vi "Main VI open close.vi"() -> ()   [LabVIEW 2022 SP3]
panel:
  in  "stop":bool
  in  "GO Button":bool
  in  "Enum":enum16{"SUBVI1", "SUBVI2", "SUBVI3"}(ring)
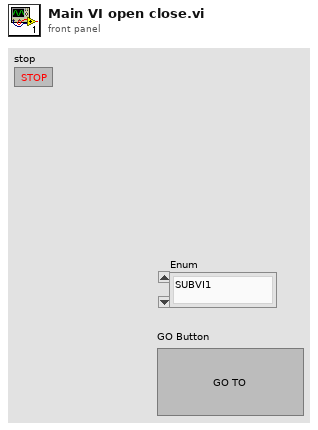
[diagram p1: front panel]
types:
  T1 = enum32{"Invalid", "Standard", "Closed", "Hidden", "Minimized", "Maximized"}
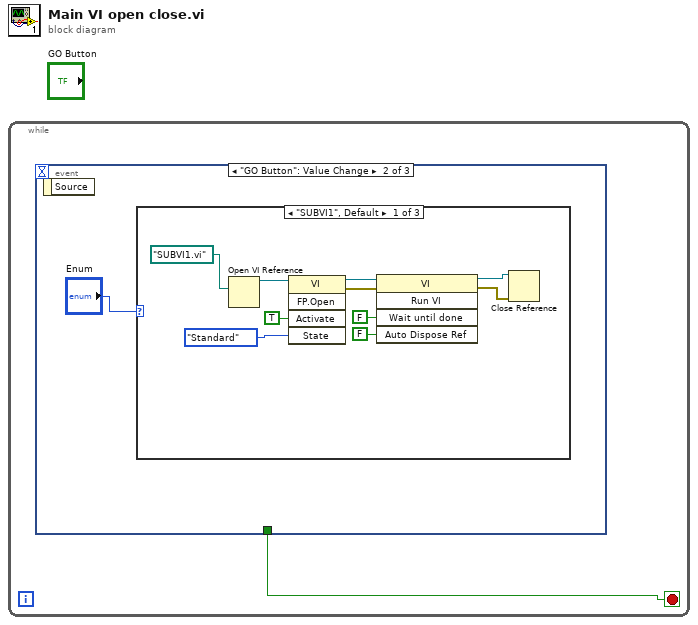
[diagram p0: block diagram]
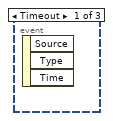
[diagram p2: hidden frame]
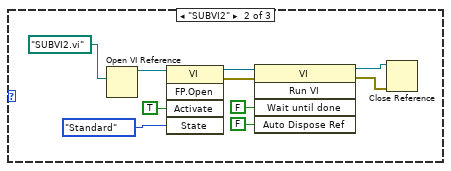
[diagram p3: hidden frame]
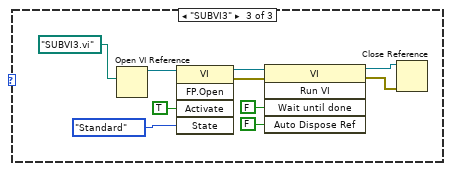
[diagram p4: hidden frame]
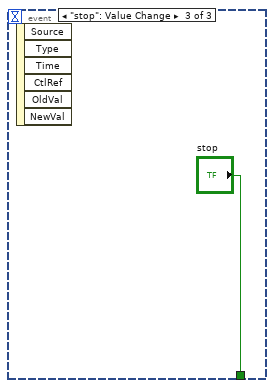
[diagram p5: hidden frame]
diagram:
  n1 = while {
    stop <- w1 stop-if-true
    n2 = event shown="[1] \"GO Button\": Value Change" {
      selector: _ -> [_ _ _]
      dyn-events: _ -> [_ _ _]
      timeout: _ -> [_ _ _]
      tunnel: [_ _ "stop"] -> w1
      event Timeout {
        n3 = event-data() -> ()  [unwired: 1 in, 3 out]
      }
      event "GO Button": Value Change {
        n4 = event-data() -> ()  [unwired: 1 in, 1 out]
        n5 = case shown="\"SUBVI1\", Default" "Enum" {
          frame "SUBVI1", Default {
            n6 = Open VI Reference(vi path=path "SUBVI1.vi") -> (vi reference=w11:refnum<vi>)  [unwired: 5 in, 1 out]
            n7 = invoke class="VI" method="FP.Open"(reference=w11, "Activate"=TRUE ("Activate?"), "State"=T1."Standard") -> (reference out=w8:refnum<vi>, error out=w7:errorcluster)  [unwired: 2 in, 3 out]
            n8 = invoke class="VI" method="Run VI"(reference=w8, error in=w7, "Wait until done"=FALSE ("Wait Until Done"), "Auto Dispose Ref"=FALSE ("Auto Dispose Reference")) -> (reference out=w4:refnum<vi>, error out=w3:errorcluster)  [unwired: 1 in, 3 out]
            n9 = Close Reference(reference=w4, error in (no error)=w3) -> ()  [unwired: 1 out]
          }
          frame "SUBVI2" {
            n10 = Open VI Reference(vi path=path "SUBVI2.vi") -> (vi reference=w21:refnum<vi>)  [unwired: 5 in, 1 out]
            n11 = invoke class="VI" method="FP.Open"(reference=w21, "Activate"=TRUE ("Activate?"), "State"=T1."Standard") -> (reference out=w18:refnum<vi>, error out=w17:errorcluster)  [unwired: 2 in, 3 out]
            n12 = invoke class="VI" method="Run VI"(reference=w18, error in=w17, "Wait until done"=FALSE ("Wait Until Done"), "Auto Dispose Ref"=FALSE ("Auto Dispose Reference")) -> (reference out=w14:refnum<vi>, error out=w13:errorcluster)  [unwired: 1 in, 3 out]
            n13 = Close Reference(reference=w14, error in (no error)=w13) -> ()  [unwired: 1 out]
          }
          frame "SUBVI3" {
            n14 = Open VI Reference(vi path=path "SUBVI3.vi") -> (vi reference=w31:refnum<vi>)  [unwired: 5 in, 1 out]
            n15 = invoke class="VI" method="FP.Open"(reference=w31, "Activate"=TRUE ("Activate?"), "State"=T1."Standard") -> (reference out=w28:refnum<vi>, error out=w27:errorcluster)  [unwired: 2 in, 3 out]
            n16 = invoke class="VI" method="Run VI"(reference=w28, error in=w27, "Wait until done"=FALSE ("Wait Until Done"), "Auto Dispose Ref"=FALSE ("Auto Dispose Reference")) -> (reference out=w24:refnum<vi>, error out=w23:errorcluster)  [unwired: 1 in, 3 out]
            n17 = Close Reference(reference=w24, error in (no error)=w23) -> ()  [unwired: 1 out]
          }
        }
      }
      event "stop": Value Change {
        n18 = event-data() -> ()  [unwired: 1 in, 6 out]
      }
    }
  }
